vi "Unflatten From Message String.vi"(11 "Message":string) -> (0 "error out":errorcluster, 3 "Log Packet":T1)   [LabVIEW 2019, in "Network Sink.lvlib" / "LogEventMessageProtocol.lvclass"]
uses:
  <vilib>/gpm_packages/@cs/event-logger/Source/Network Sink/LogEventMessageProtocol/LogEventMessageProtocol.lvclass
  <vilib>/gpm_packages/@cs/event-logger/Source/Composed Log/Types/Log Packet.ctl
  <vilib>/gpm_packages/@cs/event-logger/Source/Composed Log/Types/Log Level.ctl
  <vilib>/gpm_packages/@cs/event-logger/Source/Composed Log/Composed Log.lvlib
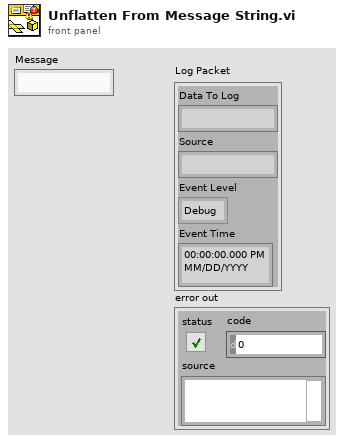
[diagram p1: front panel]
types:
  T1 = typedef "Composed Log.lvlib/Log Packet.ctl" = cluster{"Data To Log":string, "Source":string, "Event Level":T2, "Event Time":timestamp}
  T2 = typedef "Composed Log.lvlib/Log Level.ctl" = enum16{"Debug", "Info", "Warning", "Error", "Critical"}
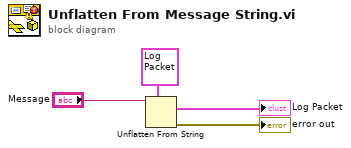
[diagram p0: block diagram]
diagram:
  n1 = Unflatten From String(type=T1 {"Data To Log"="", "Source"="", "Event Level"=enum."Debug", "Event Time"=timestamp(0 s since 1904-01-01)} ("Log Packet"), binary string="Message") -> (value=→"Log Packet":T1, error out=→"error out":errorcluster)  [unwired: 3 in, 1 out]
